vi "Divide.vi"(8 "error in (no error)":errorcluster, 10 "Divider":dbl, 11 "Data2D in":refnum<class "Data2D.lvclass">) -> (0 "error out":errorcluster, 3 "Data2D out":refnum<class "Data2D.lvclass">)   [LabVIEW 2014, in "Data2D.lvclass"]
uses:
  Data2D.lvclass
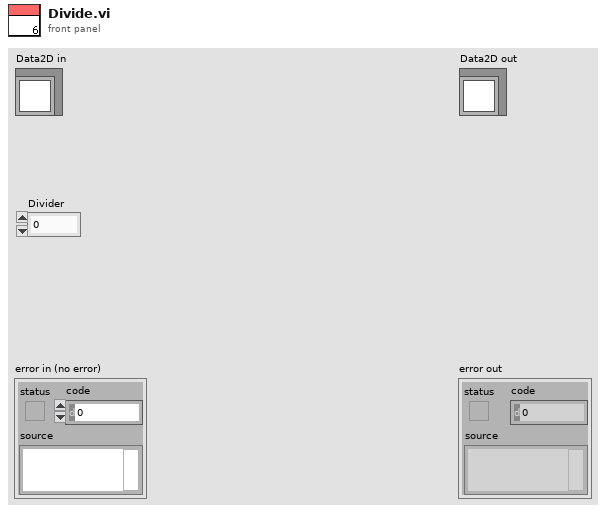
[diagram p1: front panel]
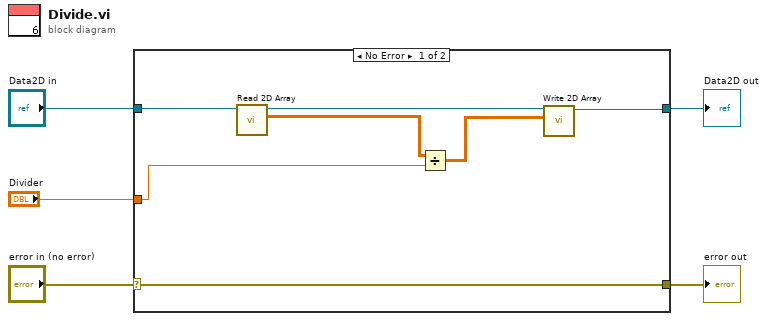
[diagram p0: block diagram]
diagram:
  n1 = case shown="No Error" "error in (no error)" {
    selector: "error in (no error)" -> [w12 w14]
    tunnel: [w12 w14] -> w4
    tunnel: [w9 w13] -> w2
    tunnel: "Data2D in" -> [w11 w13]
    tunnel: "Divider" -> [w6 _]
    frame No Error {
      n2 = call "Read 2D Array.vi"("Data2D in"=w11) -> ("2D Array"=w8:dbl[][], "Data2D out"=w10:refnum<class "Data2D.lvclass">)  [unwired: 8 in, 1 out]
      n3 = Divide(x=w8, y=w6) -> (x/y=w7:dbl[][])
      n4 = call "Write 2D Array.vi"("2D Array"=w7, "Data2D in"=w10) -> ("Data2D out"=w9:refnum<class "Data2D.lvclass">)  [unwired: 8 in, 1 out]
    }
    frame Error {
    }
  }
  "error out" <- w4
  "Data2D out" <- w2
